vi "Interlocks Example.vi"() -> ()   [LabVIEW 2022 SP3]
uses:
  Interlocks/Interlocks.lvlib
panel:
  in  "Override Interlocks?":bool
  in  "V5":bool
  in  "V3":bool
  in  "MFC1":dbl min=0.0 max=10.0 step=0.1 format="%.1f"
  in  "V1":bool
  in  "V2":bool
  in  "V4":bool
  in  "Stop":bool
  # "Instructions:\nRun this VI and toggle the valves to see the interlocks enable or disable the\ncontrols accordingly to the expressions defined in the Interlocks.ini file as:"
  # "Expressions supported:\nAND:          and | && | &\nOR:           or | '||' | '|'\nNOT:          not | !\nEQUAL:        ==\nNOT EQUAL:    !=\nLESS THAN:    <\nGREATER THAN: >\nLTE:          <=\nGTE:          >=\nPARENTHESES:  (..)\nLITERAL:      Boolean | DBL | I32 | U32\nIDENTIFIER:   [A-Za-z_][A-Za-z0-9_]*"
  # "[<variable_name>]\n<expression>"
  # "If the expression is evaluated to True or is empty, the control is Enabled.\nOtherwise the control is Disabled and grayed out.\nSet Override Interlocks? to True, to enable all controls."
  # "Gas\nInlet"
  # "[V2]\nnot V1 and\n(V4 or V5)"
  # "[V1]\nnot V2 and\n(V4 or V5)"
  # "[V3]\nV1 or V2"
  # "Example Expression:\nV1 and not V2 and (MFC1 > 4.5 or V3) or V5"
  # "; Interlocks.ini\n; [<variable_name>]\n; <expression>\n;------------------\n[V1]\nnot V2 and (V4 or V5)\n\n[V2]\nnot V1 and (V4 or V5)\n\n[V3]\nV1 or V2\n\n[MFC1]\nV3 and (V1 or V2)\n\n[V4]\nnot (V1 or V2) and\nnot V5 or MFC1 > 0.5\n\n[V5]\nnot (V1 or V2) and\nnot V4 or MFC1 > 0.5"
  # "Water\nInlet"
  # "[MFC1]\nV3 and (V1 or V2)"
  # "[V4]\nnot (V1 or V2) and\nnot V5 or \nMFC1 > 0.5"
  # "Return"
  # "[V5]\nnot (V1 or V2) and\nnot V4 or\nMFC1 > 0.5"
  # "Drain"
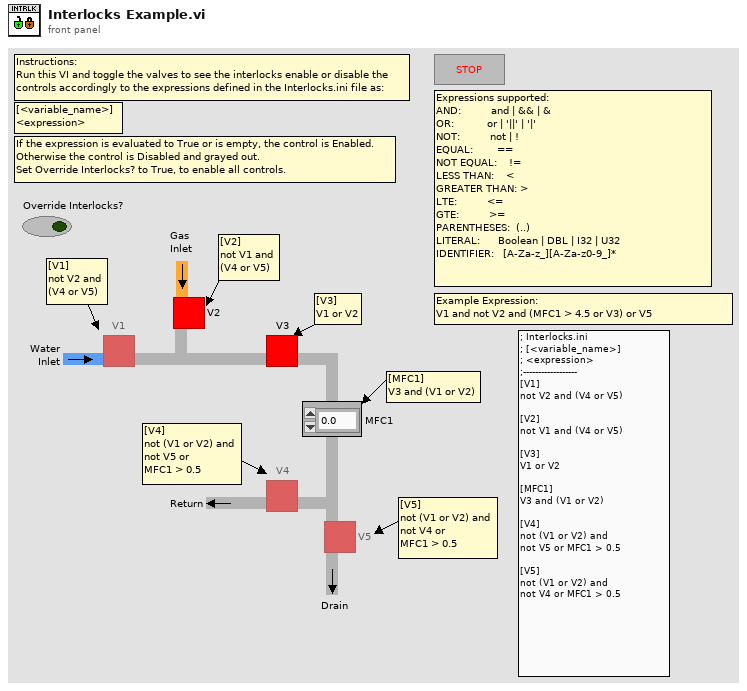
[diagram p1: front panel]
types:
  T1 = enum32{"invalid app kind", "Development System", "Run Time System", "Student Edition", "Embedded LabVIEW", "Evaluation", "Custom"}
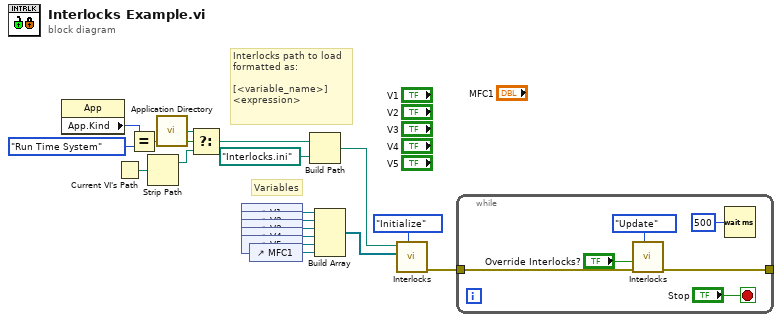
[diagram p0: block diagram]
diagram:
  # "Interlocks path to load\nformatted as:\n\n[<variable_name>]\n<expression>"
  # "Variables"
  n1 = property class="App"() -> ("App.Kind"=w7:T1)  [unwired: 2 in, 2 out]
  n2 = Current VI's Path() -> (path=w4:path)
  n3 = Equal?(x=w7, y=T1."Run Time System") -> (x = y?=w5:bool)
  n4 = Strip Path(path=w4) -> (stripped path=w1:path)  [unwired: 1 out]
  n5 = call <vilib>:"Application Directory.vi"() -> ("Application Directory"=w3:path)
  n6 = Select(t=w3, s=w5, f=w1) -> (s? t:f=w2:path)
  n7 = control-ref of="V1"() -> (w15:refnum<vi>)
  n8 = control-ref of="V2"() -> (w14:refnum<vi>)
  n9 = control-ref of="V3"() -> (w13:refnum<vi>)
  n10 = control-ref of="V4"() -> (w12:refnum<vi>)
  n11 = control-ref of="V5"() -> (w11:refnum<vi>)
  n12 = control-ref of="MFC1"() -> (w10:refnum<vi>)
  n13 = Build Path(base path=w2, name or relative path=path "Interlocks.ini") -> (appended path=w8:path)
  n14 = Build Array(w15, w14, w13, w12, w11, w10) -> (w16:refnum<vi>[])
  n15 = call "Interlocks.vi"("Action"=enum16{"Initialize", "Update"}."Initialize", "Variables"=w16, "Interlocks (.ini)"=w8) -> ("error out"=w17:errorcluster)  [unwired: 8 in]
  n16 = while {
    tunnel: w17 -> [w23]
    tunnel: [w21] -> _
    stop <- "Stop" stop-if-true
    n17 = call "Interlocks.vi"("Action"=enum16{"Initialize", "Update"}."Update", "error in (no error)"=w23, "Override? (F)"="Override Interlocks?") -> ("error out"=w21:errorcluster)  [unwired: 8 in]
    n18 = Wait (ms)(milliseconds to wait=u32 500) -> ()  [unwired: 1 out]
  }
